vi "rqc Random Number Generator.vi"(7 "reset":bool, 9 "initial seed":u32=4294967295 caption="seed", 10 "rndGen.parameters":T1={"value type"=enum."constant", "constant"=0, "num of levels"=0, "levels values"=[0, 0, 0, 0]}) -> (2 "DAC random level":u8)   [LabVIEW 2018]
uses:
  Custom Controls/rqc Random Generator.parameters.ctl
  Custom Controls/rqc Random Generator.value type.ctl
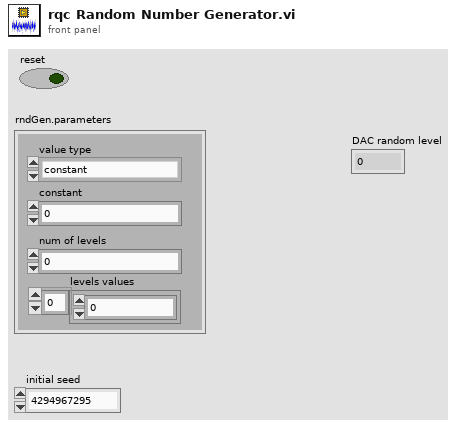
[diagram p1: front panel]
types:
  T1 = typedef "rqc Random Generator.parameters.ctl" = cluster{"value type":T2, "constant":u16, "num of levels":u16, "levels values":u16[]}
  T2 = typedef "rqc Random Generator.value type.ctl" = enum16{"random value", "constant"}
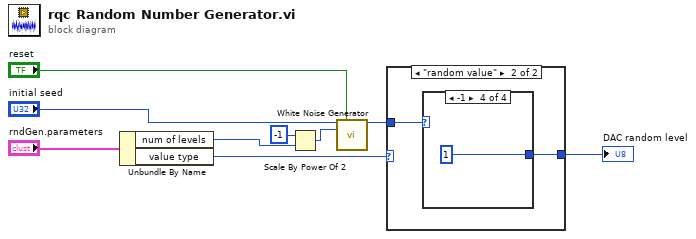
[diagram p0: block diagram]
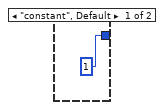
[diagram p2: hidden frame]
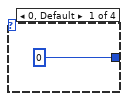
[diagram p3: hidden frame]
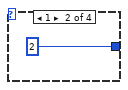
[diagram p4: hidden frame]
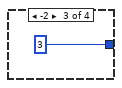
[diagram p5: hidden frame]
diagram:
  n1 = Unbundle By Name("rndGen.parameters") -> ("num of levels"=w5:u16, "value type"=w4:T2)
  n2 = Scale By Power Of 2(n=i16 -1, x=w5) -> (x*2^n=w7:u16)
  n3 = call "White Noise Generator"("seed"="initial seed", "reset"="reset", "amplitude"=w7) -> ("white noise out"=w9:i16)  [unwired: 12 in]
  n4 = case shown="\"random value\"" w4 {
    tunnel: w9 -> [_ w12]
    tunnel: [u8 1 ("index") w11] -> w1
    frame "constant", Default {
    }
    frame "random value" {
      n5 = case shown="-1" w12 {
        tunnel: [u8 0 ("index") u8 2 ("index") u8 3 ("index") u8 1 ("index")] -> w11
        frame 0, Default {
        }
        frame 1 {
        }
        frame -2 {
        }
        frame -1 {
        }
      }
    }
  }
  "DAC random level" <- w1
